vi "dl.vi"() -> ()   [LabVIEW 2025]
uses:
  <vilib>/Instr/_visa.llb/VISA Configure Serial Port (Instr).vi
panel:
  out "KONDENSATOR":dbl(slide) scale=2.8..3.3
  in  "?":bool
  in  "ILOŒÆ D¯ULI":dbl
  out "OSTATNI LOG":string
  out "LOGI":string[](array[string])
  in  "KONTRAST":dbl(knob) scale=0.0..1000.0
  in  "?":bool
  in  "?":bool
  in  "?":bool
  out "KONDENSATOR":dbl(graph)
  in  "stop":bool
  out "AKTUALNA WARTOŒÆ":dbl
  out "REZYSTOR":dbl(graph)
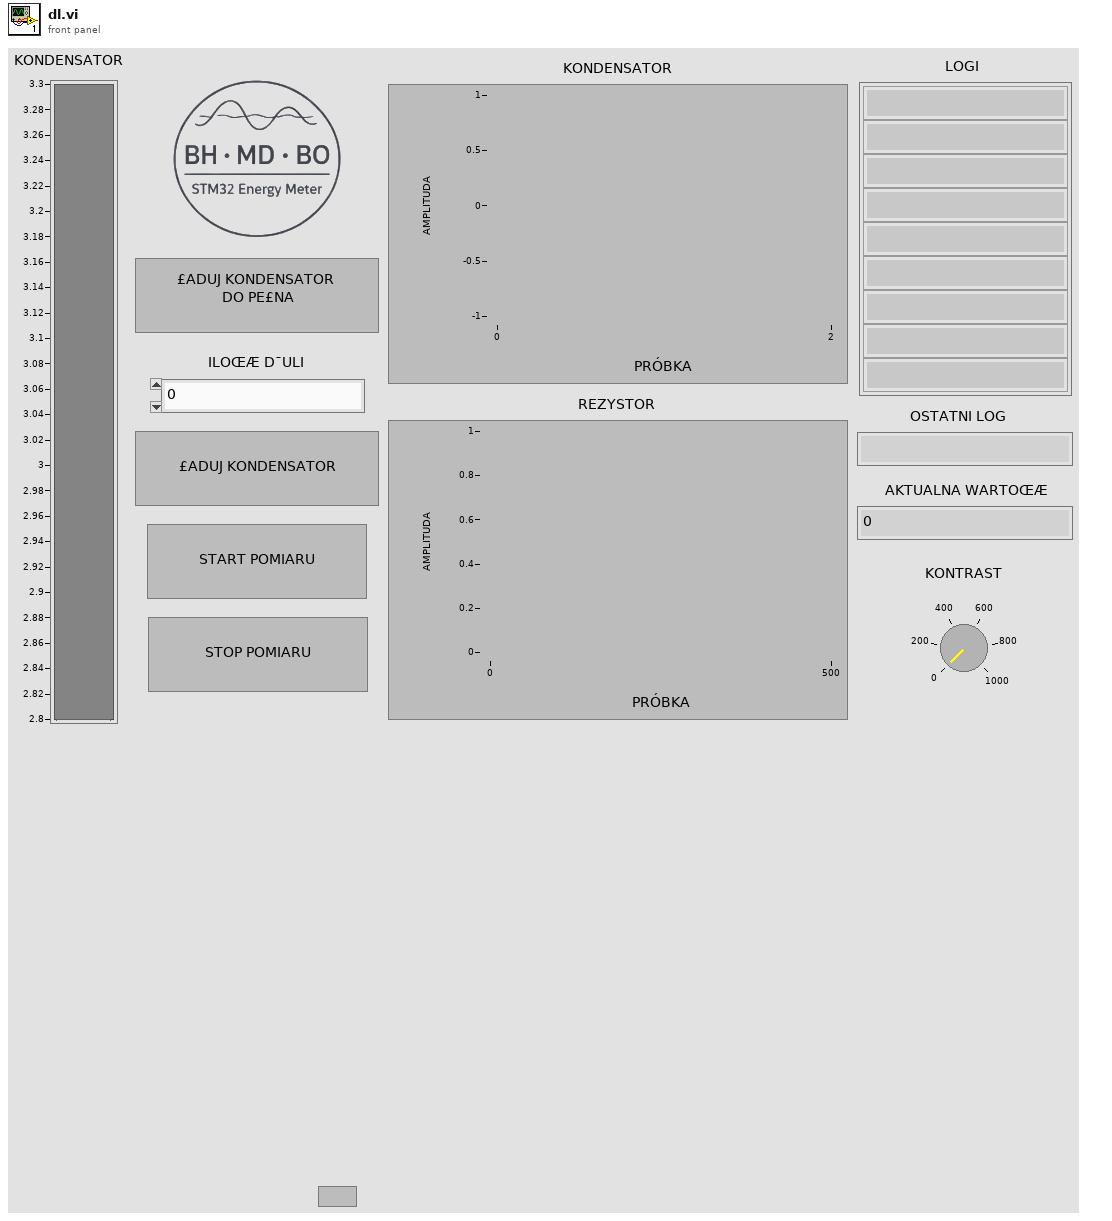
[diagram p1: front panel]
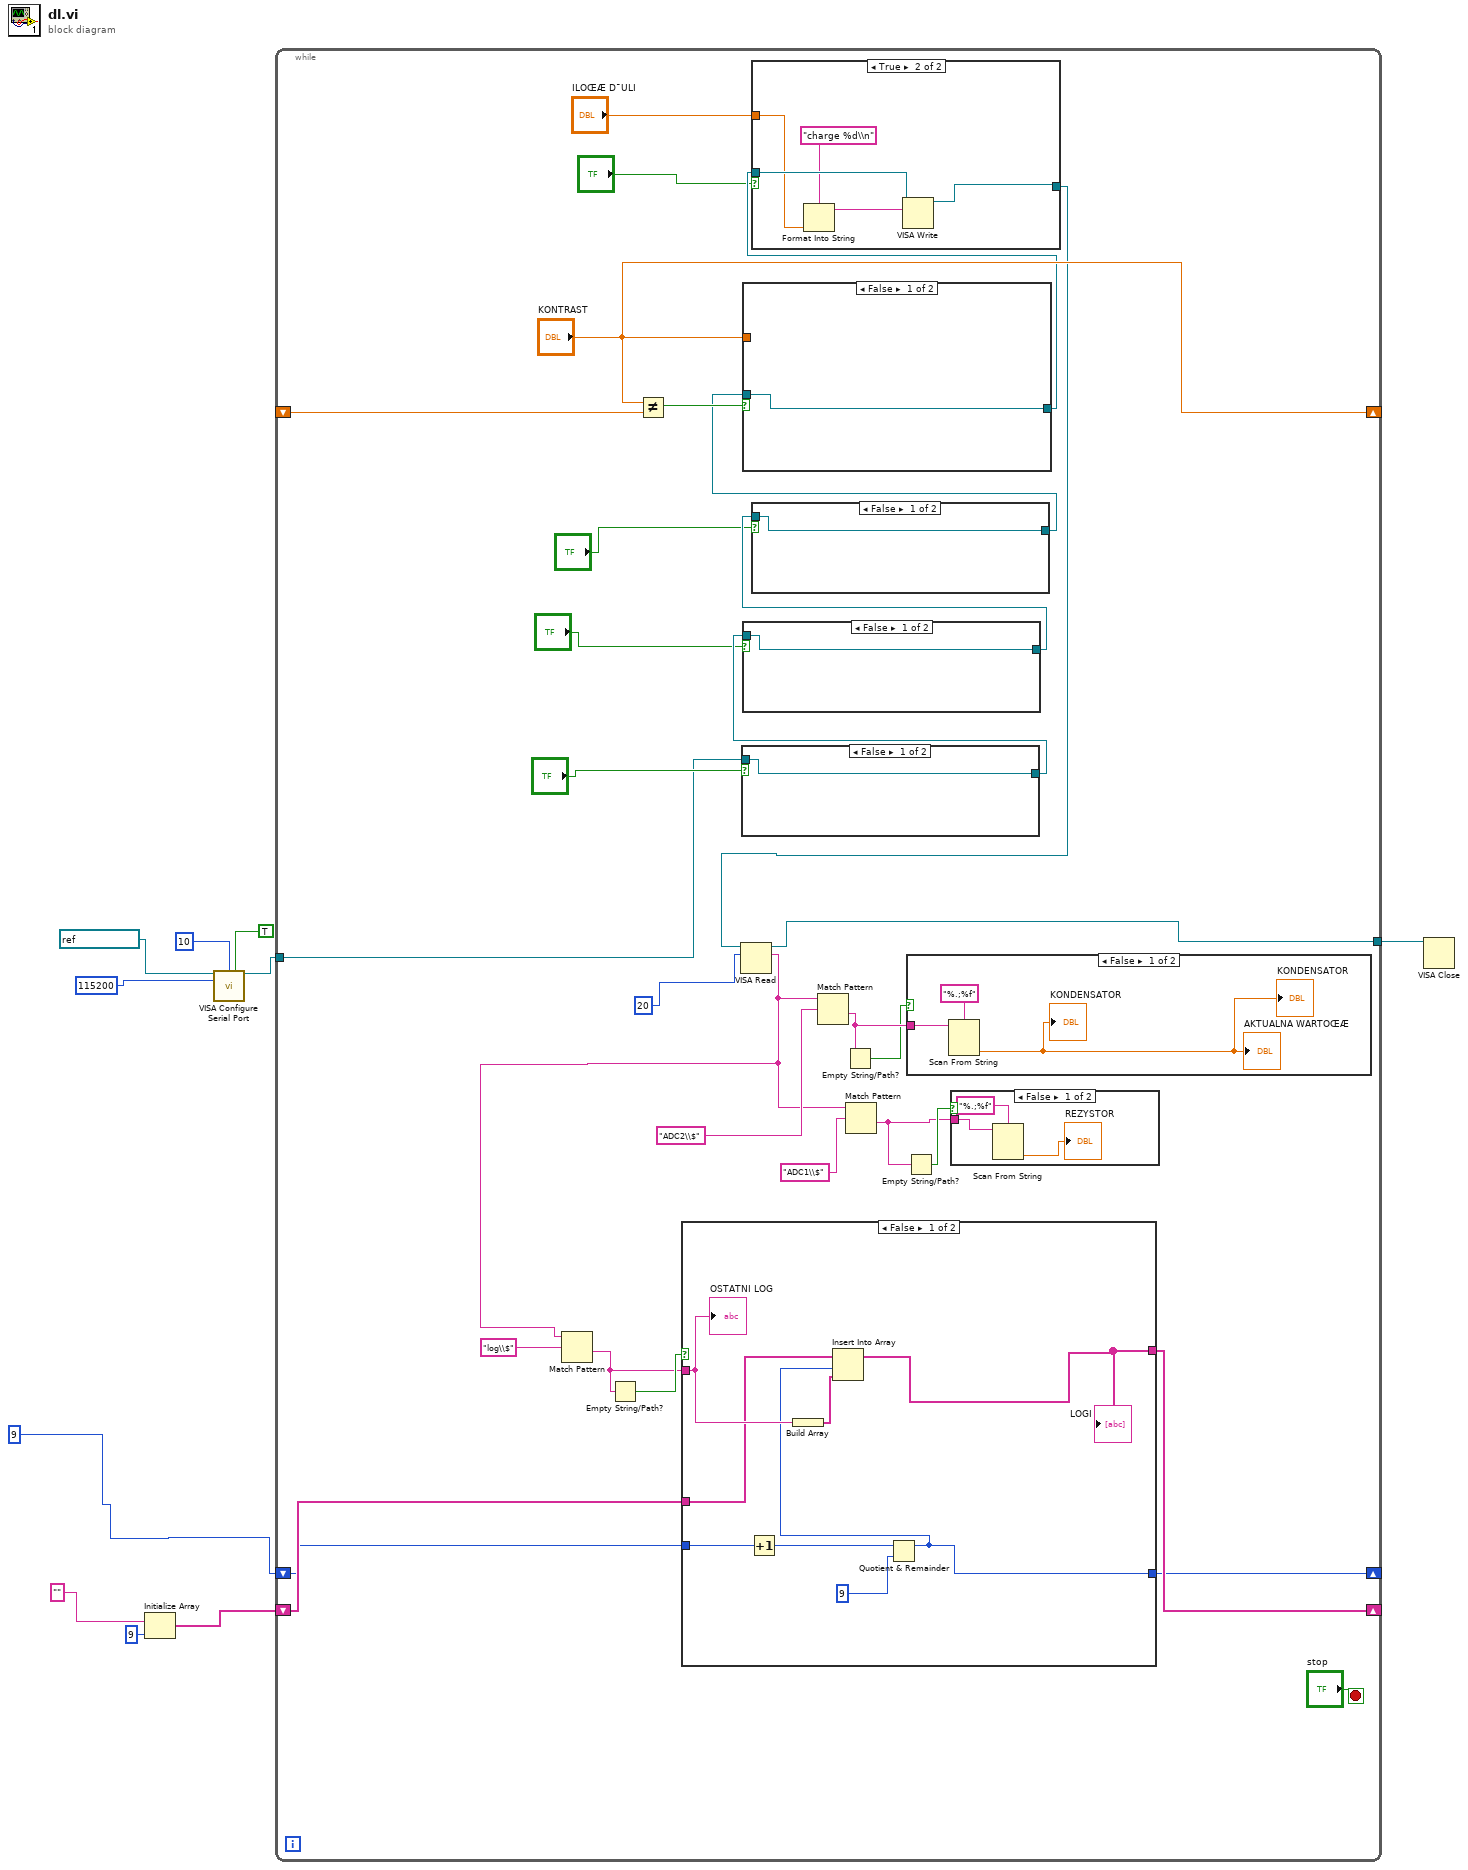
[diagram p0: block diagram]
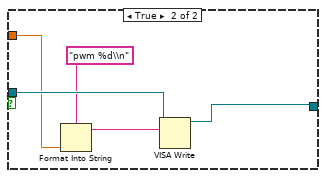
[diagram p4: hidden frame]
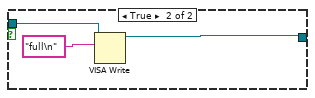
[diagram p5: hidden frame]
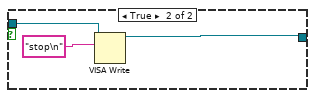
[diagram p6: hidden frame]
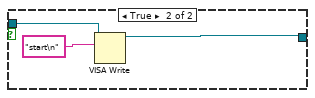
[diagram p7: hidden frame]
diagram:
  n1 = Initialize Array("", 9 ("dimension size")) -> (w2:string[])
  n2 = call-poly "VISA Configure Serial Port"("VISA resource name"=refnum<visa-resource-name> "COM10", "termination char\n(0xA = '\\n' = LF)"=u8 10 ("termination char\n(0xA = '\\n' = LF)"), "Enable Termination\nChar (T)"=TRUE ("Enable Termination\nChar (T)"), "baud rate (9600)"=u32 115200) -> ("VISA resource name out"=w5:refnum<visa-resource-name>)  [unwired: 10 in, 1 out]
  n3 = while {
    tunnel: w5 -> [w19]
    tunnel: [w39] -> w6
    shift-right: ["KONTRAST"] -> _
    shift-left: _ -> [w25]
    shift-right: [w20] -> _
    shift-left: w2 -> [w17]
    shift-right: [w15] -> _
    shift-left: 9 ("y") -> [w16]
    stop <- "stop" stop-if-true
    n4 = Not Equal?(x="KONTRAST", y=w25) -> (x != y?=w27:bool)
    n5 = case shown="False" "?" {
      tunnel: w19 -> [w72 w75]
      tunnel: [w72 w73] -> w31
      frame False {
      }
      frame True {
        n6 = VISA Write(VISA resource name=w75, write buffer="start\n") -> (VISA resource name out=w73:refnum<visa-resource-name>)  [unwired: 1 in, 2 out]
      }
    }
    n7 = case shown="False" "?" {
      tunnel: w31 -> [w68 w71]
      tunnel: [w68 w69] -> w29
      frame False {
      }
      frame True {
        n8 = VISA Write(VISA resource name=w71, write buffer="stop\n") -> (VISA resource name out=w69:refnum<visa-resource-name>)  [unwired: 1 in, 2 out]
      }
    }
    n9 = case shown="False" "?" {
      tunnel: w29 -> [w64 w67]
      tunnel: [w64 w65] -> w26
      frame False {
      }
      frame True {
        n10 = VISA Write(VISA resource name=w67, write buffer="full\n") -> (VISA resource name out=w65:refnum<visa-resource-name>)  [unwired: 1 in, 2 out]
      }
    }
    n11 = case shown="False" w27 {
      tunnel: w26 -> [w58 w63]
      tunnel: [w58 w62] -> w13
      tunnel: "KONTRAST" -> [_ w60]
      frame False {
      }
      frame True {
        n12 = Format Into String(format string="pwm %d\\n", w60) -> (resulting string=w61:string)  [unwired: 2 in, 1 out]
        n13 = VISA Write(VISA resource name=w63, write buffer=w61) -> (VISA resource name out=w62:refnum<visa-resource-name>)  [unwired: 1 in, 2 out]
      }
    }
    n14 = case shown="True" "?" {
      tunnel: w13 -> [w42 w47]
      tunnel: [w42 w46] -> w14
      tunnel: "ILOŒÆ D¯ULI" -> [_ w44]
      frame False {
      }
      frame True {
        n15 = Format Into String(format string="charge %d\\n", w44) -> (resulting string=w45:string)  [unwired: 2 in, 1 out]
        n16 = VISA Write(VISA resource name=w47, write buffer=w45) -> (VISA resource name out=w46:refnum<visa-resource-name>)  [unwired: 1 in, 2 out]
      }
    }
    n17 = VISA Read(VISA resource name=w14, byte count=u32 20) -> (VISA resource name out=w39:refnum<visa-resource-name>, read buffer=w18:string)  [unwired: 1 in, 2 out]
    n18 = Match Pattern(string=w18, regular expression="log\\$") -> (after substring=w21:string)  [unwired: 1 in, 3 out]
    n19 = Empty String/Path?(string/path=w21) -> (empty?=w23:bool)
    n20 = case shown="False" w23 {
      tunnel: w21 -> [w55 _]
      tunnel: [w48 w57] -> w20
      tunnel: w17 -> [w52 w57]
      tunnel: w16 -> [w50 w56]
      tunnel: [w49 w56] -> w15
      frame False {
        n21 = Increment(x=w50) -> (x+1=w51:i32)
        n22 = Build Array(w55) -> (w54:string[])
        n23 = Quotient & Remainder(x=w51, y=9) -> (x-y*floor(x/y)=w49:i32)  [unwired: 1 out]
        n24 = Insert Into Array(array=w52, index=w49, new element=w54) -> (w48:string[])
        "LOGI" <- w48
        "OSTATNI LOG" <- w55
      }
      frame True {
      }
    }
    n25 = Match Pattern(string=w18, regular expression="ADC2\\$") -> (after substring=w34:string)  [unwired: 1 in, 3 out]
    n26 = Empty String/Path?(string/path=w34) -> (empty?=w33:bool)
    n27 = Match Pattern(string=w18, regular expression="ADC1\\$") -> (after substring=w35:string)  [unwired: 1 in, 3 out]
    n28 = Empty String/Path?(string/path=w35) -> (empty?=w36:bool)
    n29 = case shown="False" w33 {
      tunnel: w34 -> [w77 _]
      frame False {
        n30 = Scan From String(format string="%.;%f", input string=w77) -> (output 1=→"AKTUALNA WARTOŒÆ" →"KONDENSATOR" →"KONDENSATOR":dbl)  [unwired: 3 in, 3 out]
      }
      frame True {
      }
    }
    n31 = case shown="False" w36 {
      tunnel: w35 -> [w79 _]
      frame False {
        n32 = Scan From String(format string="%.;%f", input string=w79) -> (output 1=→"REZYSTOR":dbl)  [unwired: 3 in, 3 out]
      }
      frame True {
      }
    }
  }
  n33 = VISA Close(VISA resource name=w6) -> ()  [unwired: 1 in, 1 out]
